vi "Normalize by Max AbsVal.vi"(1 "Y":dbl[](array[numeric])) -> (0 "Ynorm":dbl[](array[numeric]))   [LabVIEW 2020]
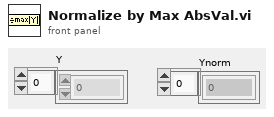
[diagram p1: front panel]
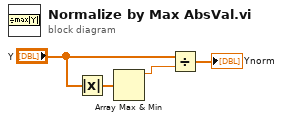
[diagram p0: block diagram]
diagram:
  n1 = Absolute Value(x="Y") -> (abs(x)=w2:dbl[])
  n2 = Array Max & Min(array=w2) -> (max value=w1:dbl)  [unwired: 3 out]
  n3 = Divide(x="Y", y=w1) -> (x/y=→"Ynorm":dbl[])
